vi "Cervical_Detect_InnerROI_SubVI.vi"(8 "error in":errorcluster, 11 "Raw Image":T2) -> (0 "error out":errorcluster, 1 "ROI Descriptor":T1 {"Contours"."Type" items=["No Selection", "Point", "Line", "Rectangle", "Oval", "Polygon", "Freehand Region", "Annulus", "Unused2", "Unused3", "Broken Line", "Freehand Line", "Rotated Rectangle"]}, 2 "Predicted Mask":T2(plugin-control), 3 "Raw Frame Out":T2(plugin-control))   [LabVIEW 2021]
uses:
  <vilib>/vision/Image Controls.llb/IMAQ Image.ctl
  <vilib>/vision/NI_Vision_Development_Module.lvlib
panel:
  # "83"
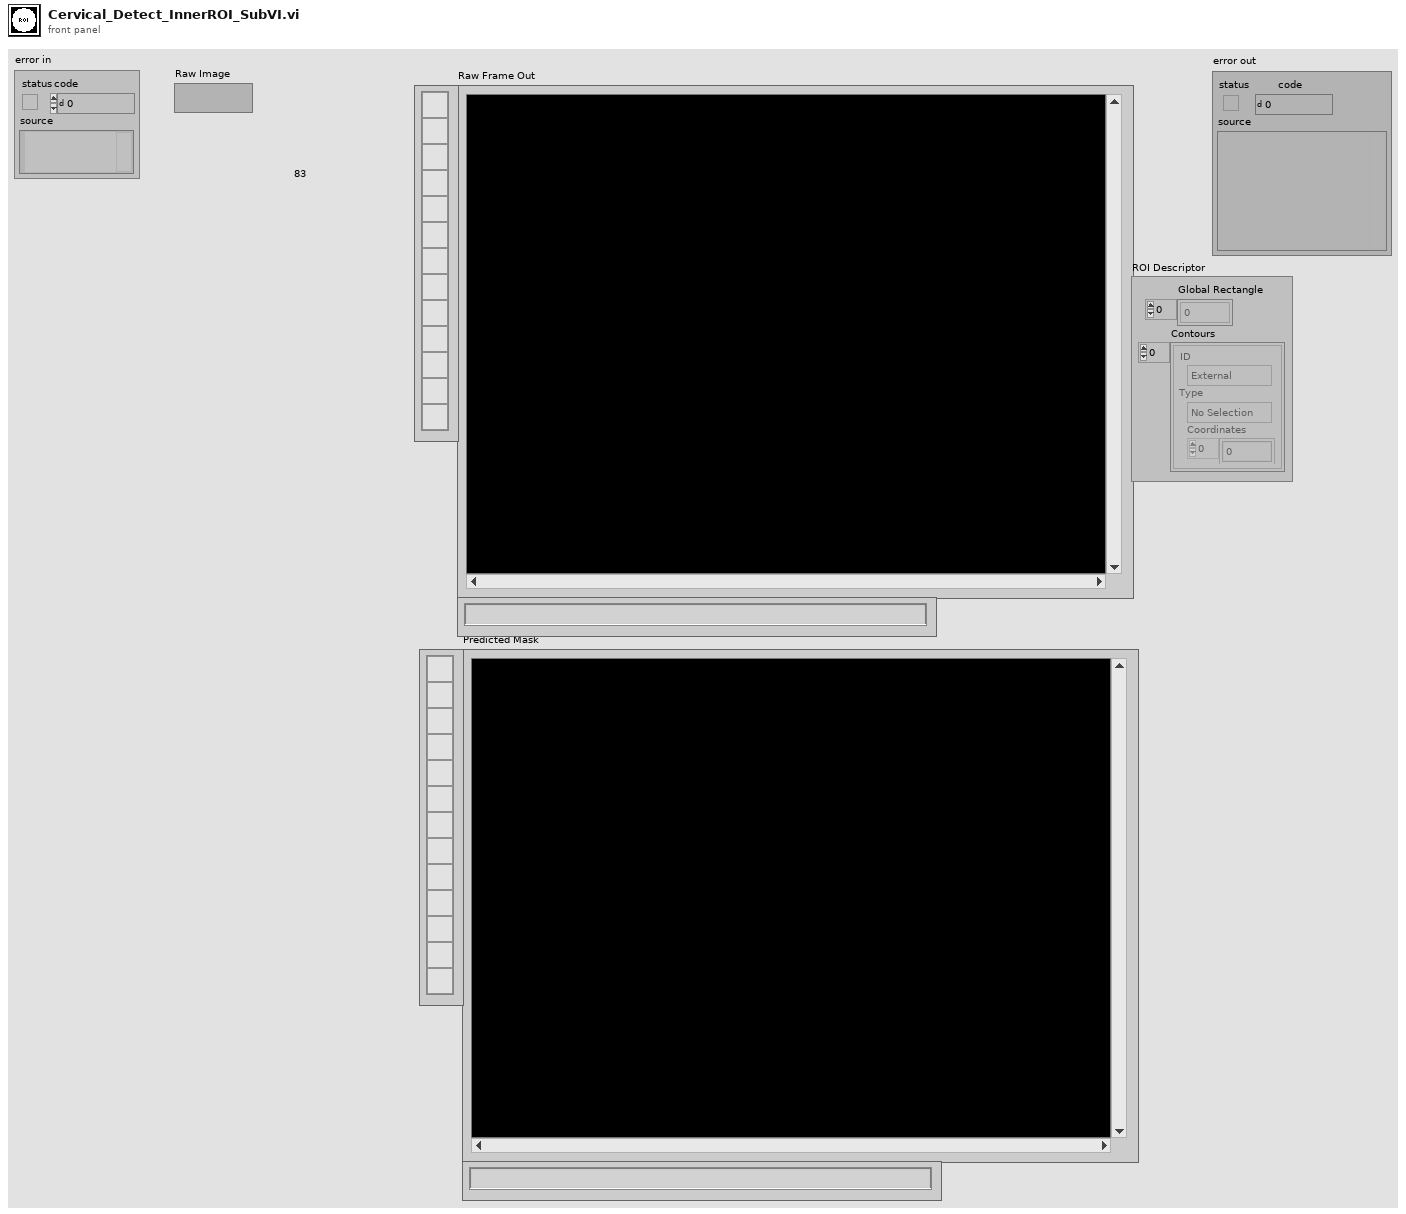
[diagram p1: front panel]
types:
  T1 = typedef "ROI Descriptor" = cluster{"Global Rectangle":i32[], "Contours":cluster{"ID":enum32{"External", "Internal"}, "Type":u32, "Coordinates":i32[]}[]}
  T2 = typedef "IMAQ Image.ctl" = refnum<image>
  T3 = typedef "Image Type" = u32
  T4 = enum32{"AutoM", "Close", "Dilate", "Erode", "Gradient", "Gradient out", "Gradient in", "Hit miss", "Open", "PClose", "POpen", "Thick", "Thin"}
  T5 = cluster{"Pos. X":i32, "Pos. Y":i32, "Radius":i32, "Core Area":i32}[]
  T6 = cluster{"Pos. X":i32, "Pos. Y":i32, "Radius":i32, "Core Area":i32}
  T7 = typedef "IMAQ Circle" = cluster{"Center X":i32, "Center Y":i32, "Inner Radius":i32, "Outer Radius":i32, "Start Angle":dbl, "End Angle":dbl}
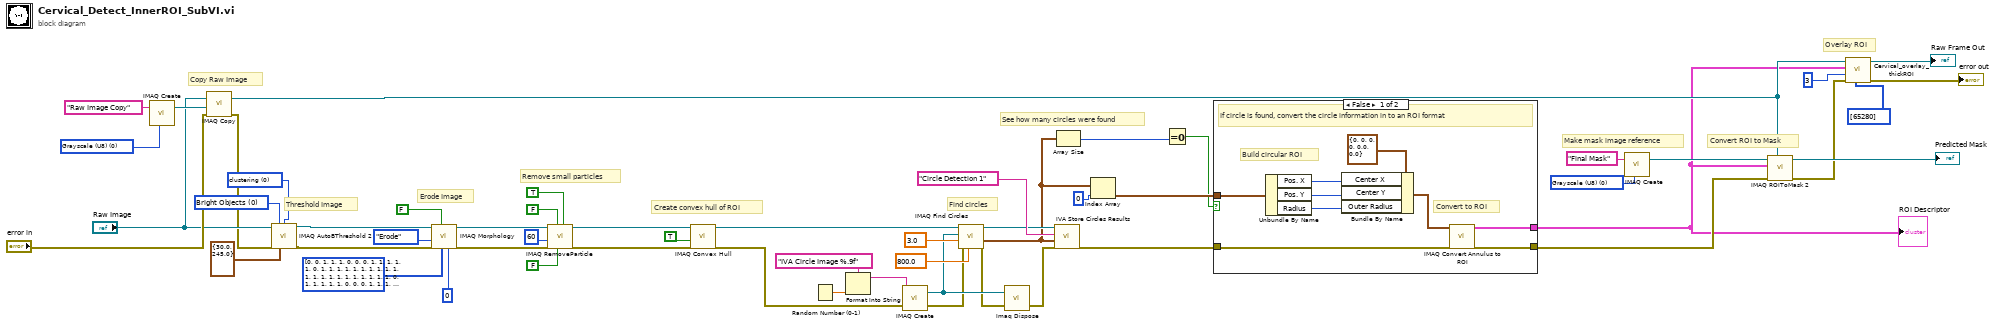
[diagram p0: block diagram]
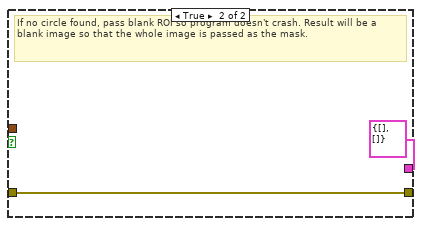
[diagram p2: hidden frame]
diagram:
  w14 = 0 items=["clustering", "entropy", "metric", "moments", "inter-class variance"] ("Method")
  w13 = u32 0 items=["Bright Objects", "Dark Objects"] ("Look For")
  w26 = T3 0 items=["Grayscale (U8)", "Grayscale (I16)", "Grayscale (SGL)", "Complex (CSG)", "RGB (U32)", "HSL (U32)", "RGB (U64)", "Grayscale (U16)"] ("Image Type")
  w31 = T3 0 items=["Grayscale (U8)", "Grayscale (I16)", "Grayscale (SGL)", "Complex (CSG)", "RGB (U32)", "HSL (U32)", "RGB (U64)", "Grayscale (U16)"] ("Image Type")
  # "See how many circles were found"
  # "Overlay ROI"
  # "Convert ROI to Mask"
  # "Make mask image reference"
  # "Copy Raw Image"
  # "Find circles"
  # "Create convex hull of ROI"
  # "Remove small particles"
  # "Erode Image"
  # "Threshold Image"
  n1 = call "IMAQ Create"("Image Name"="Raw Image Copy", "Image Type"=w31) -> ("New Image"=w30:T2)  [unwired: 2 in, 2 out]
  n2 = call "IMAQ Copy"("error in (no error)"="error in", "Image Dst"=w30, "Image Src"="Raw Image") -> ("error out"=w16:errorcluster, "Image Dst Out"=w7:T2)  [unwired: 3 in]
  n3 = call "IMAQ AutoBThreshold 2"("Image Src"="Raw Image", "Look For (Bright Objects)"=w13, "Method (clustering)"=w14, "error in (no error)"=w16, "Threshold Limits"=cluster{"Lower value":sgl, "Upper value":sgl} {"Lower value"=30.0, "Upper value"=245.0}) -> ("Image Dst Out"=w18:T2, "error out"=w17:errorcluster)  [unwired: 3 in, 6 out]
  n4 = call "IMAQ Morphology"("Number of iterations (1)"=0, "Structuring Element"=i32[][] [[0, 0, 1, 1, 1, 0, 0], [0, 1, 1, 1, 1, 1, 0], [1, 1, 1, 1, 1, 1, 1], [1, 1, 1, 1, 1, 1, 1], [1, 1, 1, 1, 1, 1, 1], [0, 1, 1, 1, 1, 1, 0], [0, 0, 1, 1, 1, 0, 0]], "Square/Hexa (Square)"=FALSE, "error in (no error)"=w17, "Operation"=T4."Erode", "Image Src"=w18) -> ("error out"=w11:errorcluster, "Image Dst Out"=w12:T2)  [unwired: 1 in, 3 out]
  n5 = call "IMAQ RemoveParticle"("Connectivity 4/8 (8)"=TRUE, "Low Pass/High Pass (Low)"=FALSE, "Square/Hexa (Square)"=FALSE, "error in (no error)"=w11, "Number of Erosion"=60, "Image Src"=w12) -> ("error out"=w46:errorcluster, "Image Dst Out"=w45:T2)  [unwired: 1 in, 3 out]
  n6 = call "IMAQ Convex Hull"("error in (no error)"=w46, "Connectivity 4/8 (8)"=TRUE, "Image Src"=w45) -> ("error out"=w43:errorcluster, "Image Dst Out"=w29:T2)  [unwired: 1 in, 6 out]
  n7 = Random Number (0-1)() -> (number: 0 to 1=w33:dbl)
  n8 = Format Into String(format string="IVA Circle Image %.9f" ("Image Name"), w33) -> (resulting string=w35:string)  [unwired: 2 in, 1 out]
  n9 = call "IMAQ Create"("Image Name"=w35, "error in (no error)"=w43) -> ("New Image"=w40:T2, "error out"=w39:errorcluster)  [unwired: 2 in, 1 out]
  n10 = call "IMAQ Find Circles"("Max Radius"=sgl 800.0, "error in (no error)"=w39, "Min Radius"=sgl 3.0, "Image Dst"=w40, "Image Src"=w29) -> ("error out"=w38:errorcluster, "Circles Data"=w10:T5)  [unwired: 5 out]
  n11 = call "Imaq Dispose"("Image"=w40, "error in (no error)"=w38) -> ("error out"=w37:errorcluster)  [unwired: 1 in, 3 out]
  n12 = call <vilib>:"IVA Store Circles Results.vi"("error in (no error)"=w37, "Circles Data"=w10, "Step Name"="Circle Detection 1", "Image in"=w29) -> ("error out"=w21:errorcluster)  [unwired: 7 out]
  n13 = Array Size(array=w10) -> (size(s)=w9:i32)
  n14 = Index Array(array=w10, index=0) -> (element=w22:T6)
  n15 = Equal To 0?(x=w9) -> (x = 0?=w8:bool)
  n16 = case shown="False" w8 {
    tunnel: [w61 T1 {"Global Rectangle"=[], "Contours"=[]} ("ROI Descriptor")] -> w6
    tunnel: w22 -> [w60 _]
    tunnel: w21 -> [w56 w65]
    tunnel: [w55 w65] -> w20
    frame False {
      # "Convert to ROI"
      # "Build circular ROI"
      # "If circle is found, convert the circle information in to an ROI format"
      n17 = Unbundle By Name(w60) -> ("Pos. X"=w59:i32, "Pos. Y"=w58:i32, "Radius"=w57:i32)
      n18 = Bundle By Name(cluster=T7 {"Center X"=0, "Center Y"=0, "Inner Radius"=0, "Outer Radius"=0, "Start Angle"=0.0, "End Angle"=0.0} ("Annulus"), "Center X"=w59, "Center Y"=w58, "Outer Radius"=w57) -> (w62:T7)
      n19 = call "IMAQ Convert Annulus to ROI"("error in (no error)"=w56, "Annulus"=w62) -> ("error out"=w55:errorcluster, "ROI Descriptor"=w61:T1)  [unwired: 7 in]
    }
    frame True {
      # "If no circle found, pass blank ROI so program doesn't crash. Result will be a blank image so that the whole image is passed as the mask."
    }
  }
  "ROI Descriptor" <- w6
  n20 = call "IMAQ Create"("Image Name"="Final Mask", "Image Type"=w26) -> ("New Image"=w25:T2)  [unwired: 2 in, 2 out]
  n21 = call "IMAQ ROIToMask 2"("Image Model"=w7, "error in (no error)"=w20, "ROI Descriptor"=w6, "Image"=w25) -> ("error out"=w5:errorcluster, "Image Out"=→"Predicted Mask":T2)  [unwired: 5 in, 1 out]
  n22 = call "Cervical_overlay_thickROI.vi"("Color"=u32[] [65280], "error in (no error)"=w5, "Thickness"=3, "ROI"=w6, "Image"=w7) -> ("error out"=→"error out":errorcluster, "Image Out"=→"Raw Frame Out":T2)  [unwired: 5 in]
